vi "Rodrigues (RVec To RMat).vi"(8 "error in (no error)":errorcluster, 11 "rvec":T2) -> (0 "error out":errorcluster, 3 "Rotation Matrix":T1)   [LabVIEW 2020, in "ar.lvlib"]
doc: "Convert between Axis-Angle Rotation Vec format and 3x3 Rotation Matricies using the Rodrigues' rotation formula."
uses:
  ar.lvlib
  rvec.ctl
  <vilib>/Analysis/Matrix/Datatypes/RealMatrix.ctl
  <vilib>/Analysis/Matrix/Numeric/Conversions/Array To Matrix - RA2.vi
  <vilib>/Analysis/Matrix/NI_Matrix.lvlib
  common/common.lvlib
  common/bin/gartoolkit_ar_32-1.dll
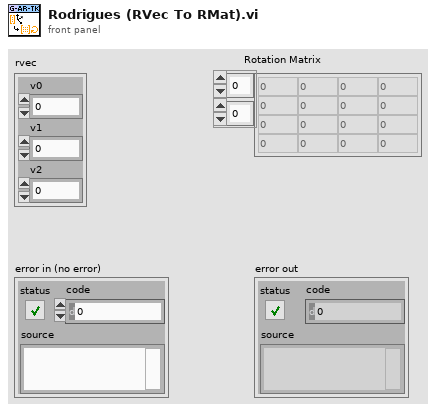
[diagram p1: front panel]
types:
  T1 = typedef "NI_Matrix.lvlib/RealMatrix.ctl" = dbl[][]
  T2 = typedef "ar.lvlib/rvec.ctl" = cluster{"v0":dbl, "v1":dbl, "v2":dbl}
  T3 = cluster{"m 0,0":dbl, "m 0,1":dbl, "m 0,2":dbl, "m 1,0":dbl, "m 1,1":dbl, "m 1,2":dbl, "m 2,0":dbl, "m 2,1":dbl, "m 2,2":dbl}
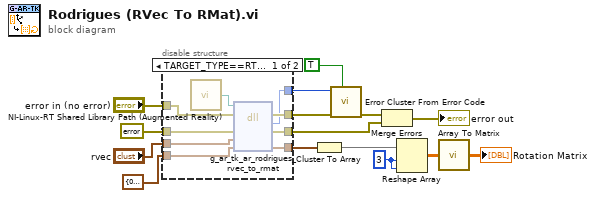
[diagram p0: block diagram]
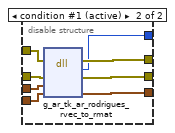
[diagram p2: hidden frame]
diagram:
  w12 = 3 ("dimension size")
  n1 = disable-structure shown="TARGET_TYPE==RT&&OS==Linux" {
    disable-tunnel: "error in (no error)" -> [w23 w32]
    disable-tunnel: errorcluster {"status"=FALSE, "code"=0, "source"=""} ("error constant") -> [w22 w31]
    disable-tunnel: "rvec" -> [w21 w30]
    disable-tunnel: T3 {"m 0,0"=0.0, "m 0,1"=0.0, "m 0,2"=0.0, "m 1,0"=0.0, "m 1,1"=0.0, "m 1,2"=0.0, "m 2,0"=0.0, "m 2,1"=0.0, "m 2,2"=0.0} ("Matrix") -> [w20 w29]
    disable-tunnel: [w19 w28] -> w5
    disable-tunnel: [w18 w27] -> w4
    disable-tunnel: [w17 w26] -> w3
    disable-tunnel: [w16 w25] -> w2
    frame condition #0 {
      n2 = call "NI-Linux-RT Shared Library Path (Augmented Reality).vi"() -> ("Path"=w24:path)
      n3 = dll-call lib="?" fn="g_ar_tk_ar_rodrigues_rvec_to_rmat" ("g_ar_toolkit.*.*:g_ar_tk_image_copy")(path in=w24, error in=w23, "error_cluster"=w22, "rvec"=w21, "rmat"=w20) -> (error out=w19:errorcluster, w18:i32, "error_cluster"=w17:errorcluster, "rmat"=w16:T3)  [unwired: 2 in, 1 out]
    }
    frame condition #1 (active) {
      n4 = dll-call lib="C:/serenial/lib/g-augmented-reality-toolkit/LabVIEW/common/bin/gartoolkit_ar_*-1.*" fn="g_ar_tk_ar_rodrigues_rvec_to_rmat" ("g_ar_toolkit.*.*:g_ar_tk_image_copy")(error in=w32, "error_cluster"=w31, "rvec"=w30, "rmat"=w29) -> (error out=w28:errorcluster, w27:i32, "error_cluster"=w26:errorcluster, "rmat"=w25:T3)  [unwired: 3 in, 1 out]
    }
  }
  n5 = Cluster To Array(cluster=w2) -> (array=w13:dbl[])
  n6 = call <vilib>:"Error Cluster From Error Code.vi"("show call chain? (False)"=TRUE, "error in (no error)"=w5, "error code (0)"=w4) -> ("error out"=w15:errorcluster)  [unwired: 6 in]
  n7 = Merge Errors(w15, w3) -> (→"error out":errorcluster)
  n8 = Reshape Array(w13, w12, w12) -> (w11:dbl[][])
  n9 = call-poly <vilib>:"Array To Matrix.vi"("Real 2D Array"=w11) -> ("Real Matrix"=→"Rotation Matrix":T1)
